vi "cluster_to_image.vi"(1 "CLUSTER":i32[][](array[numeric])) -> (0 "Image":T1(plugin-control))   [LabVIEW 2018]
panel:
  out "Tableau":u32[][](array[numeric])
  in  "LUT":u32[](array[colorbox])=[16711680, 6618880, 16860, 16774930, 16711844, 16744192, 4849919, 1985280, 6372155, 1230335]
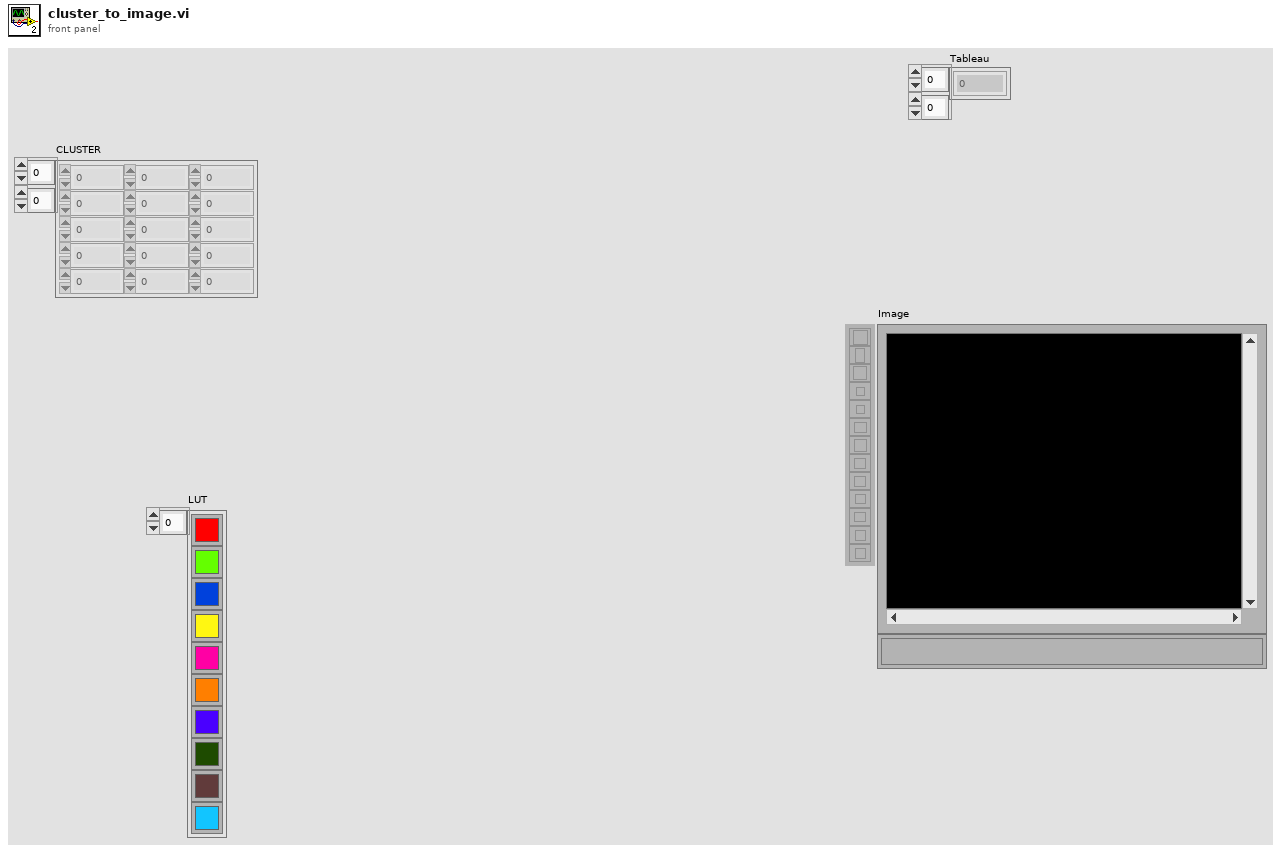
[diagram p1: front panel]
types:
  T1 = typedef "IMAQ Image.ctl" = refnum<image>
  T2 = typedef "Image Type" = u32
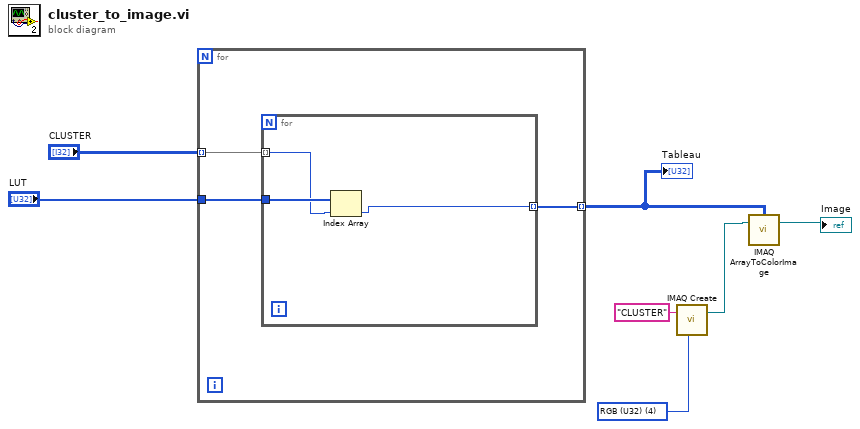
[diagram p0: block diagram]
diagram:
  w3 = T2 4 items=["Grayscale (U8)", "Grayscale (I16)", "Grayscale (SGL)", "Complex (CSG)", "RGB (U32)", "HSL (U32)", "RGB (U64)", "Grayscale (U16)"] ("Image Type")
  n1 = for {
    tunnel: "CLUSTER" -> [w10] mode=indexing
    tunnel: "LUT" -> [w9]
    tunnel: [w8] -> w5 mode=indexing
    n2 = for {
      tunnel: w10 -> [w12] mode=indexing
      tunnel: w9 -> [w13]
      tunnel: [w11] -> w8 mode=indexing
      n3 = Index Array(array=w13, index=w12) -> (element=w11:u32)
    }
  }
  "Tableau" <- w5
  n4 = call "IMAQ Create"("Image Name"="CLUSTER", "Image Type"=w3) -> ("New Image"=w2:T1)  [unwired: 3 in, 1 out]
  n5 = call "IMAQ ArrayToColorImage"("Image Pixels (U32)"=w5, "Image"=w2) -> ("Image Out"=→"Image":T1)  [unwired: 3 in, 1 out]
